vi "DataTreeCtrl buildFileNode.vi"(6 "Extension pattern":string="*.tdms", 7 "Item":T2={"Left Cell String"="", "Child Text"=[], "Child Tag"="", "Item Indent"=1, "Child Only?"=TRUE, "Glyph Index"=0}, 11 "RootPath":path) -> (2 "FileName":string[](array[string]), 3 "TreeItems":T1(array[cluster]))   [LabVIEW 2018, in "DataTreeCtrl.lvclass"]
uses:
  DataTreeCtrl.lvclass
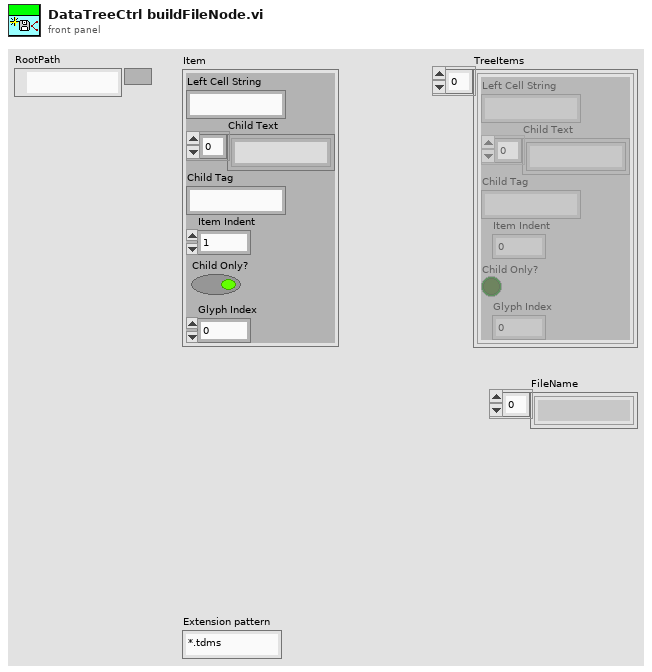
[diagram p1: front panel]
types:
  T1 = cluster{"Left Cell String":string, "Child Text":string[], "Child Tag":string, "Item Indent":i32, "Child Only?":bool, "Glyph Index":i32}[]
  T2 = cluster{"Left Cell String":string, "Child Text":string[], "Child Tag":string, "Item Indent":i32, "Child Only?":bool, "Glyph Index":i32}
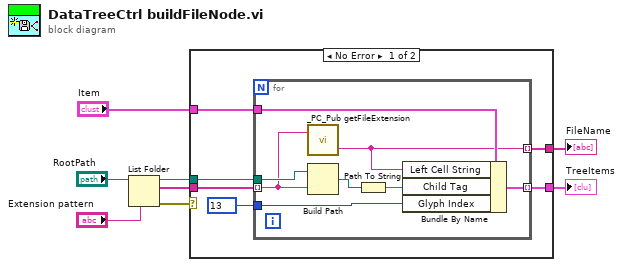
[diagram p0: block diagram]
diagram:
  n1 = List Folder(path="RootPath", pattern="Extension pattern") -> (path out=w3:path, filenames=w5:string[], error out=w6:errorcluster)  [unwired: 2 in, 1 out]
  n2 = case shown="No Error" w6 {
    tunnel: [w14 _] -> w2
    tunnel: w5 -> [w13 _]
    tunnel: "Item" -> [w11 _]
    tunnel: w3 -> [w10 _]
    tunnel: [w9 _] -> w1
    frame No Error {
      n3 = for {
        tunnel: w13 -> [w18] mode=indexing
        tunnel: [w22] -> w14 mode=indexing
        tunnel: 13 -> [w21]
        tunnel: w11 -> [w20]
        tunnel: w10 -> [w19]
        tunnel: [w15] -> w9 mode=indexing
        n4 = call "_PC_Pub getFileExtension.vi"("Input"=w18) -> ("FileName"=w15:string)  [unwired: 1 in, 1 out]
        n5 = Build Path(base path=w19, name or relative path=w18) -> (appended path=w17:path)
        n6 = Path To String(path=w17) -> (string=w16:string)
        n7 = Bundle By Name(cluster=w20, "Left Cell String"=w15, "Child Tag"=w16, "Glyph Index"=w21) -> (w22:T2)
      }
    }
    frame Error {
    }
  }
  "TreeItems" <- w2
  "FileName" <- w1
